vi "CalculateCoincidenceImage.vi"(0 "new dimension":cluster{"x":u32, "y":u32}, 1 "threshold":u32, 2 "new pixelsize x":i32, 3 "newpixelsize y":i32, 4 "ratio":bool caption="Nc", 5 "coincidence settings":T1={"length [µs]"=10.0, "delayed channel"=0, "center peak (µs)"=0.6, "lateral peaks"=2} {"lateral peaks" min=2 max=10 step=2; "center peak (µs)" format="%.2f"; "length [µs]" format="%.2f"}) -> (6 "result":dbl[][](array[numeric]) format="%.2f")   [LabVIEW 2009]
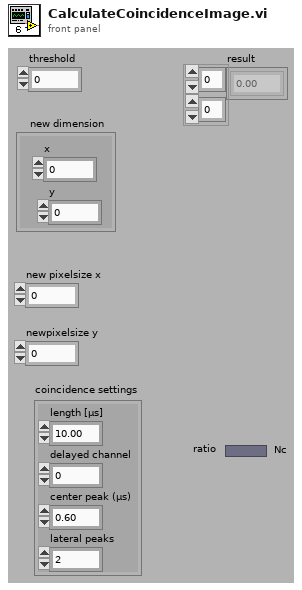
[diagram p1: front panel]
types:
  T1 = cluster{"length [µs]":dbl, "delayed channel":u8, "center peak (µs)":dbl, "lateral peaks":u32}
  T2 = cluster{"origin (ns)":dbl, "offset (ns)":dbl, "histogram":u32[]}
  T3 = typedef "ImageSettings.ctt" = cluster{"Start Position (µm)":cluster{"x":dbl, "y":dbl, "z":dbl}, "End Position (µm)":cluster{"x":dbl, "y":dbl, "z":dbl}, "Image Resolution (nm/pixel)":cluster{"x":dbl, "y":dbl, "z":dbl}, "Image Size (µm)":cluster{"x":dbl, "y":dbl, "z":dbl}, "Image Size (pixel)":cluster{"x":u32, "y":u32, "z":u32}, "Time Resolution\n(ms/pixel)":dbl, "1st Axis":u16, "2nd Axis":u16, "Retrace":bool, "Estimated Time":string}
  T4 = cluster{"origin (ns)":dbl, "offset (ns)":dbl, "histogram":u32[]}[]
  T5 = cluster{"router":u8[], "macro times":dbl[], "micro times":u16[], "invalid":dbl[], "gap":dbl[]}
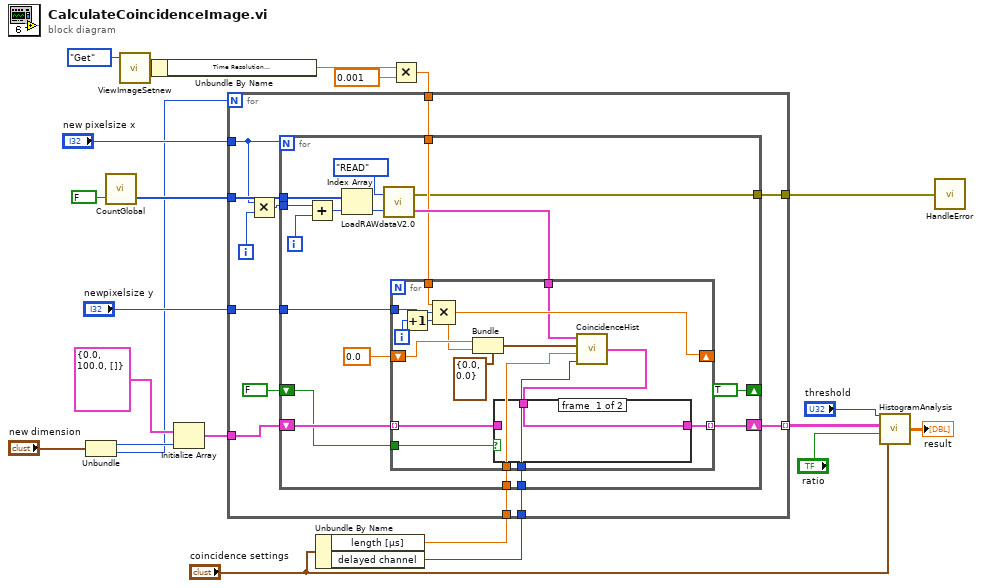
[diagram p0: block diagram]
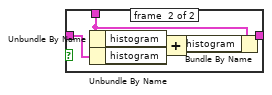
[diagram p2: hidden frame]
diagram:
  n1 = Unbundle("new dimension") -> ("x"=w7:u32, "y"=w6:u32)
  n2 = call "CountGlobal.vi"("changed?"=FALSE) -> ("count out"=w12:i32[])  [unwired: 2 in]
  n3 = call "ViewImageSetnew.vi"("action"=enum16{"Display", "change", "Get", "Set"}."Get" ("Enum")) -> ("Image Settings"=w16:T3)  [unwired: 2 in]
  n4 = Unbundle By Name(w16) -> ("Time Resolution\n(ms/pixel)"=w17:dbl)
  n5 = Initialize Array(T2 {"origin (ns)"=0.0, "offset (ns)"=100.0, "histogram"=[]} ("coincidence histogram"), w7) -> (w14:T4)
  n6 = Unbundle By Name("coincidence settings") -> ("length [µs]"=w10:dbl, "delayed channel"=w9:u8)
  n7 = Multiply(x=w17, y=0.001) -> (x*y=w19:dbl)
  n8 = for {
    N: w6 -> [_]
    tunnel: w12 -> [w34]
    tunnel: "new pixelsize x" -> [w27]
    tunnel: w14 -> [w31]
    tunnel: w19 -> [w30]
    tunnel: "newpixelsize y" -> [w28]
    tunnel: [w26] -> w22
    tunnel: w10 -> [w25]
    tunnel: w9 -> [w24]
    tunnel: [w23] -> w1 mode=indexing
    i -> [w32]
    n9 = Multiply(x=w27, y=w32) -> (x*y=w33:i32)
    n10 = for {
      N: w27 -> [_]
      tunnel: w34 -> [w51]
      tunnel: w33 -> [w48]
      shift-right: [w40] -> w23
      shift-left: w31 -> [w46]
      tunnel: w30 -> [w44]
      shift-right: [TRUE] -> _
      shift-left: FALSE -> [w41]
      tunnel: w28 -> [w39]
      tunnel: [w37] -> w26
      tunnel: w25 -> [w36]
      tunnel: w24 -> [w35]
      i -> [w49]
      n11 = Add(x=w48, y=w49) -> (x+y=w50:i32)
      n12 = Index Array(array=w51, index=w50) -> (element=w47:i32)
      n13 = call "LoadRAWdataV2.0.vi"("pos offset (0)"=w47, "action"=enum16{"OPEN", "READ", "CLOSE"}."READ" ("Enum")) -> ("RAW data"=w45:T5, "error out"=w37:errorcluster)
      n14 = for {
        tunnel: w46 -> [w63] mode=indexing
        tunnel: w45 -> [w56]
        tunnel: w44 -> [w60]
        shift-right: [w59] -> _
        shift-left: 0.0 ("x1 2") -> [w65]
        tunnel: w41 -> [w64]
        tunnel: [w57] -> w40 mode=indexing
        tunnel: w39 -> [w61]
        tunnel: w36 -> [w53]
        tunnel: w35 -> [w52]
        i -> [w62]
        n15 = Increment(x=w62) -> (x+1=w58:i32)
        n16 = Compound Arithmetic op=MULTIPLY(w60, w61, w58) -> (w59:dbl)
        n17 = Bundle(cluster=cluster{"x0":dbl, "x1":dbl} {"x0"=0.0, "x1"=0.0} ("range"), "x0"=w65, "x1"=w59) -> (w55:cluster{"x0":dbl, "x1":dbl})
        n18 = call "CoincidenceHist.vi"("delayed channel"=w52, "length (µs)"=w53, "range"=w55, "input rawdata"=w56) -> ("coincidence histogram"=w54:T2)
        n19 = case shown="True" w64 {
          tunnel: w63 -> [_ w73]
          tunnel: w54 -> [w67 w69]
          tunnel: [w67 w70] -> w57
          frame #0 {
          }
          frame #1 {
            n20 = Unbundle By Name(w69) -> ("histogram"=w72:u32[])
            n21 = Unbundle By Name(w73) -> ("histogram"=w71:u32[])
            n22 = Add(x=w72, y=w71) -> (x+y=w68:u32[])
            n23 = Bundle By Name(cluster=w69, "histogram"=w68) -> (w70:T2)
          }
        }
      }
    }
  }
  n24 = call "HistogramAnalysis.vi"("coincidence settings"="coincidence settings", "ratio"="ratio", "Array 2"=w1, "threshold"="threshold") -> ("Array"=→"result":dbl[][])
  n25 = call "HandleError.vi"("error in (no error)"=w22) -> ()
